vi "CalculateFlow (SubVI).vi"(11 "Regulator Values":T1) -> (3 "Flow [l/h]":dbl)   [LabVIEW 2015]
uses:
  TypeDefs/RegulatorValues.ctl
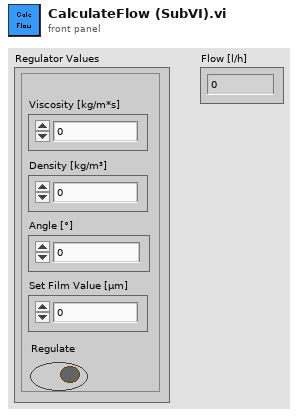
[diagram p1: front panel]
types:
  T1 = typedef "RegulatorValues.ctl" = cluster{"Viscosity [kg/m*s]":dbl, "Density [kg/m³]":dbl, "Angle [°]":dbl, "Set Film Value [µm]":dbl, "Regulate":bool}
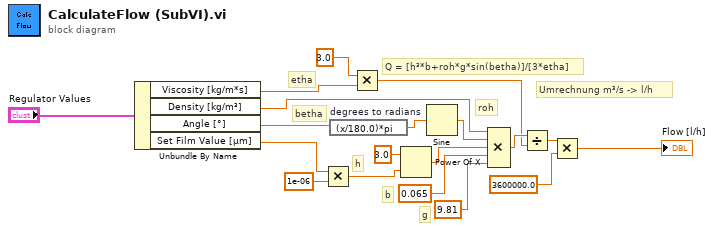
[diagram p0: block diagram]
diagram:
  # "betha"
  # "roh"
  # "h"
  # "etha"
  # "g"
  # "b"
  # "Umrechnung m³/s -> l/h"
  # "Q = [h³*b+roh*g*sin(betha)]/[3*etha]"
  n1 = Unbundle By Name("Regulator Values") -> ("Viscosity [kg/m*s]"=w1:dbl, "Density [kg/m³]"=w2:dbl, "Angle [°]"=w3:dbl, "Set Film Value [µm]"=w4:dbl)
  n2 = Multiply(x=w4, y=1e-06) -> (x*y=w8:dbl)
  n3 = expression code="(x/180.0)*pi" "degrees to radians"(w3) -> (w19:dbl)
  n4 = Multiply(x=3.0, y=w1) -> (x*y=w14:dbl)
  n5 = Power Of X(1:w8, 2:3.0 ("y")) -> (0:w10:dbl)
  n6 = Sine(x=w19) -> (sin(x)=w9:dbl)
  n7 = Compound Arithmetic op=MULTIPLY(w2, w9, w10, 0.065 ("input variable"), 9.81 ("input variable")) -> (w15:dbl)
  n8 = Divide(x=w15, y=w14) -> (x/y=w17:dbl)
  n9 = Multiply(x=w17, y=3600000.0) -> (x*y=→"Flow [l/h]":dbl)
